vi "GetTemp(SubVI).vi"(8 "error in (no error)":errorcluster, 10 "VISA resource name":refnum<visa-resource-name>="GPIB0::11::INSTR") -> (0 "error out":errorcluster, 2 "VISA resource name out":refnum<visa-resource-name>, 3 "temp":string)   [LabVIEW 2020]
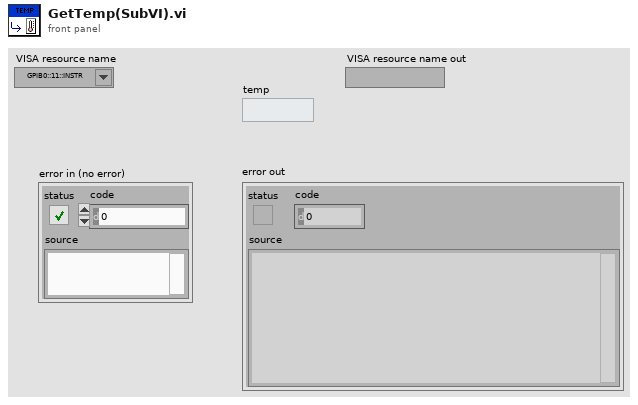
[diagram p1: front panel]
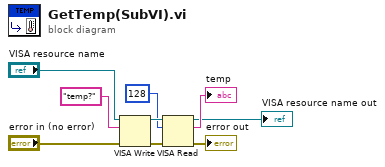
[diagram p0: block diagram]
diagram:
  n1 = VISA Write(VISA resource name="VISA resource name", write buffer="temp?", error in (no error)="error in (no error)") -> (VISA resource name out=w4:refnum<visa-resource-name>, error out=w6:errorcluster)  [unwired: 1 out]
  n2 = VISA Read(VISA resource name=w4, byte count=u32 128, error in (no error)=w6) -> (VISA resource name out=→"VISA resource name out":refnum<visa-resource-name>, read buffer=→"temp":string, error out=→"error out":errorcluster)  [unwired: 1 out]
